vi "Clear DRAM BANK1 FIFO (SubVI).vi"() -> (3 "DRAM FIFO Clear?":bool)   [LabVIEW 2015]
uses:
  <vilib>/rvi/eio/common/nirviEmuTemplateMethod_errors.vi
  <vilib>/eio/EIONode/EIONode.xnode
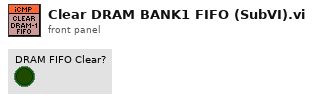
[diagram p1: front panel]
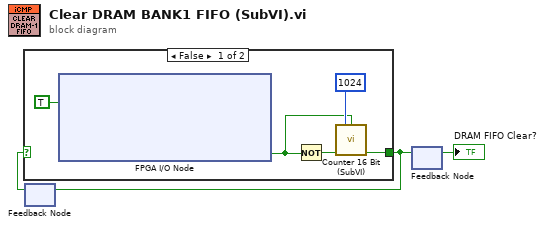
[diagram p0: block diagram]
diagram:
  n1 = feedback #1() -> (w2:bool)  [unwired: 1 in]
  n2 = case shown="False" w2 {
    selector: w2 -> [_ w9]
    tunnel: [w5 w9] -> w3
    frame False {
      n3 = xnode "FPGA I/O Node"("DRAM Bank 1\\Read"=TRUE ("DRAM Bank 0\\Read")) -> ("DRAM Bank 1\\Data_Available"=w4:bool)  [unwired: 4 in, 6 out]
      n4 = Not(x=w4) -> (.not. x?=w7:bool)
      n5 = call "Counter 16 Bit (SubVI).vi"("Max. Count"=u16 1024, "RESET"=w4, "Enable"=w7) -> ("Count End?"=w5:bool)  [unwired: 10 in, 2 out]
    }
    frame True {
    }
  }
  n6 = feedback-in #1(w3) -> ()
  n7 = feedback-in #2(w3) -> ()
  n8 = feedback #2() -> (→"DRAM FIFO Clear?":bool)  [unwired: 1 in]
